vi "Read X.vi"(2 "error in (no error)":errorcluster, 3 "Point.lvclass":refnum<class "Point.lvclass">) -> (0 "error out":errorcluster, 1 "X":dbl)   [LabVIEW 2015, in "Point.lvclass"]
uses:
  Point.lvclass
  Point.lvclass/Point.ctl
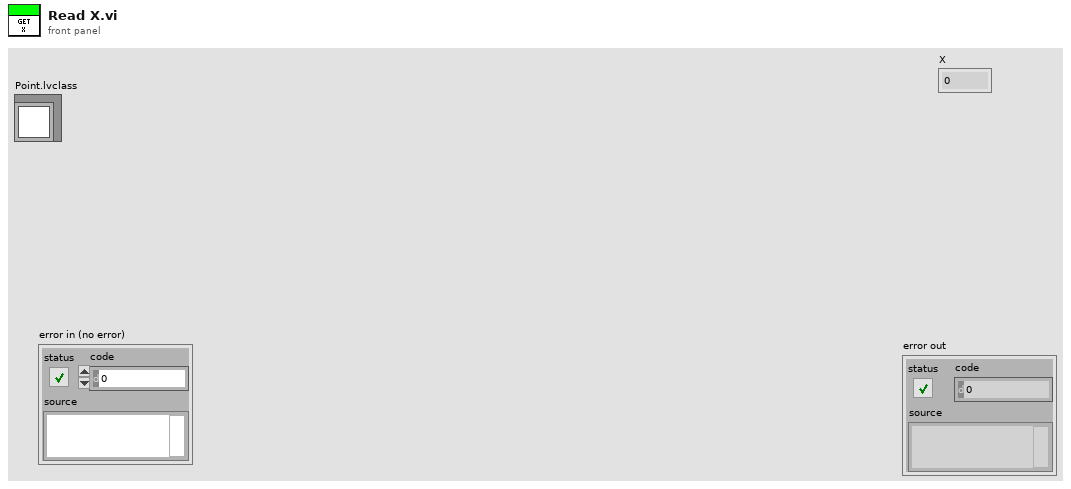
[diagram p1: front panel]
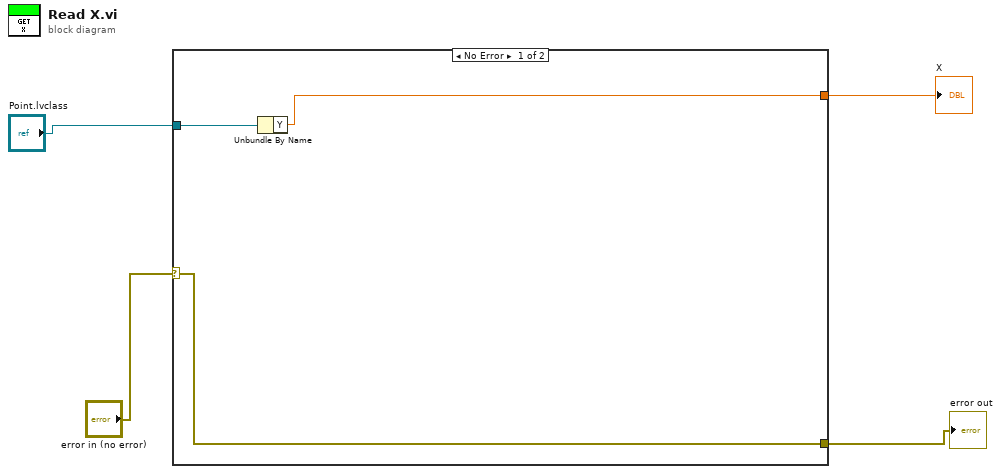
[diagram p0: block diagram]
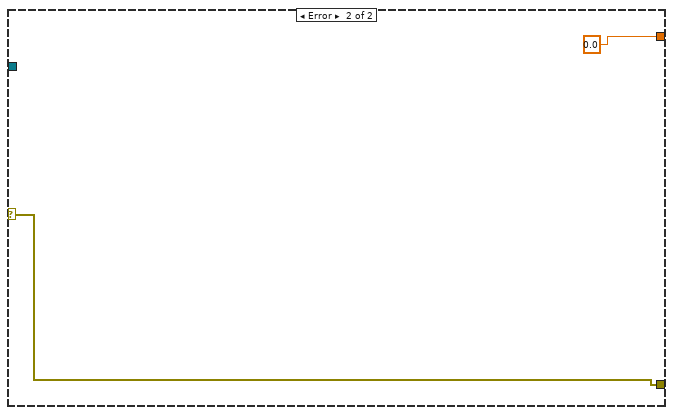
[diagram p2: hidden frame]
diagram:
  n1 = case shown="No Error" "error in (no error)" {
    selector: "error in (no error)" -> [w7 w9]
    tunnel: [w7 w9] -> w3
    tunnel: [w5 0.0] -> w2
    tunnel: "Point.lvclass" -> [w6 _]
    frame No Error {
      n2 = Unbundle By Name(w6) -> ("Y"=w5:dbl)
    }
    frame Error {
    }
  }
  "X" <- w2
  "error out" <- w3
